vi "Test_ReadItem_WrongType_ReturnTypeDefault.vi"(8 "error in (no error)":errorcluster, 11 "TestCase in":refnum<class "TestComposedLookupTable.lvclass">) -> (0 "error out":errorcluster, 3 "TestCase out":refnum<class "TestComposedLookupTable.lvclass">)   [LabVIEW 2017, in "TestComposedLookupTable.lvclass"]
uses:
  TestComposedLookupTable.lvclass
  Source/LookupTable/LookupTable.lvclass/LookupTable.ctl
  7a16431a-b6a2-4da6-80d8-a0c974427e69.vi
  045f5c79-7e11-4260-84cb-8bdda7c06bf6.vi
  Source/LookupTable/Read Table Reference.vi
  7a16431a-b6a2-4da6-80d8-a0c974427e69.vi/758d9ae7-8ccc-4b79-8ecf-981e7e60e46b.vi
  045f5c79-7e11-4260-84cb-8bdda7c06bf6.vi/3a0d2248-5a19-4a87-a56c-28eb8995d2d1.vi
  Source/LookupTable/LookupTable.lvclass
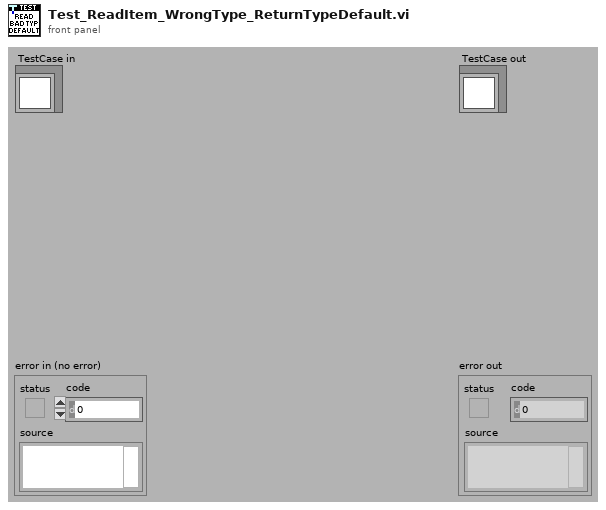
[diagram p1: front panel]
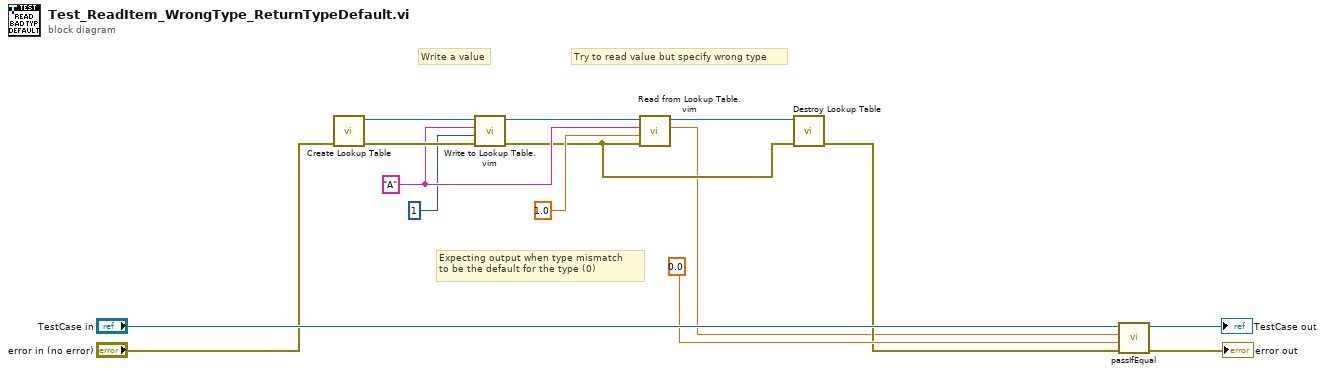
[diagram p0: block diagram]
diagram:
  w9 = "A" ("Item Name")
  # "Try to read value but specify wrong type"
  # "Write a value"
  # "Expecting output when type mismatch\nto be the default for the type (0)"
  n1 = call "Create Lookup Table.vi"("error in (no error)"="error in (no error)") -> ("error out"=w11:errorcluster, "LookupTable Reference"=w8:refnum<data-value>)  [unwired: 9 in]
  n2 = call "Write to Lookup Table.vim"("error in (no error)"=w11, "Item"=1, "Item Name"=w9, "LookupTable Reference"=w8) -> ("error out"=w4:errorcluster, "LookupTable Reference Out"=w10:refnum<data-value>)  [unwired: 5 in, 1 out]
  n3 = call "Read from Lookup Table.vim"("error in (no error)"=w4, "Type"=1.0, "Item Name"=w9, "LookupTable Reference"=w10) -> ("Value"=w1:dbl, "LookupTable Reference Out"=w7:refnum<data-value>)  [unwired: 4 in, 2 out]
  n4 = call "Destroy Lookup Table.vi"("error in (no error)"=w4, "LookupTable Reference"=w7) -> ("error out"=w2:errorcluster)  [unwired: 9 in]
  n5 = call-dynamic "passIfEqual.vi"("error in (no error)"=w2, "y"=0.0, "x"=w1, "TestCase in"="TestCase in") -> ("error out"=→"error out":errorcluster, "TestCase out"=→"TestCase out":refnum<class "TestComposedLookupTable.lvclass">)  [unwired: 6 in]
